vi "Find Object Items by Name.vi"(6 "Item Names":string[](array[string]), 7 "$Path or Item Name":string caption="Object $Path or Item Name", 8 "error in (no error)":errorcluster, 10 "Offset":i32, 11 "JSON":string) -> (0 "error out":errorcluster, 1 "<JSON>":string[](array[string]) caption="<JSON>Items", 2 "Offsets":i32[](array[numeric]))   [LabVIEW 2017, in "JSONtext.lvlib"]
doc: "Find multiple Items in a JSON Object, by item names. Output items (as JSON) are in the same order as the supplied item names. If an item is not present, then the output for that item will be an empty string."
uses:
  JSONtext.lvlib
  support/quote and escape json string 2.vi
  Offset/Find Item Locations by Path.vi
  Parsing/Parse Full Path or Item Name.vi
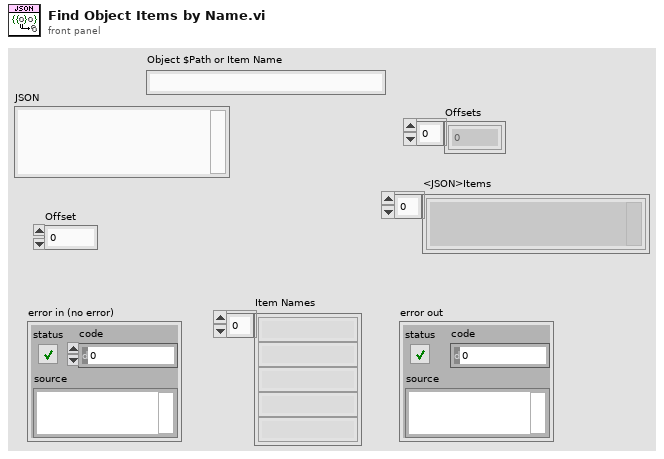
[diagram p1: front panel]
types:
  T1 = typedef "JSONtext.lvlib/Found Items.ctl" = cluster{"Item offset":i32, "Offset past Item":i32, "Name offset":i32, "Offset past Name":i32, "Found":bool, "Item Type":T2, "Item Index":i32}
  T2 = typedef "JSONtext.lvlib/Parsing State.ctl" = enum16{"Parser Error", "Object", "Array", "String", "Number/Other", "Leading Whitespace", "Object end", "Array end", "Value end"}
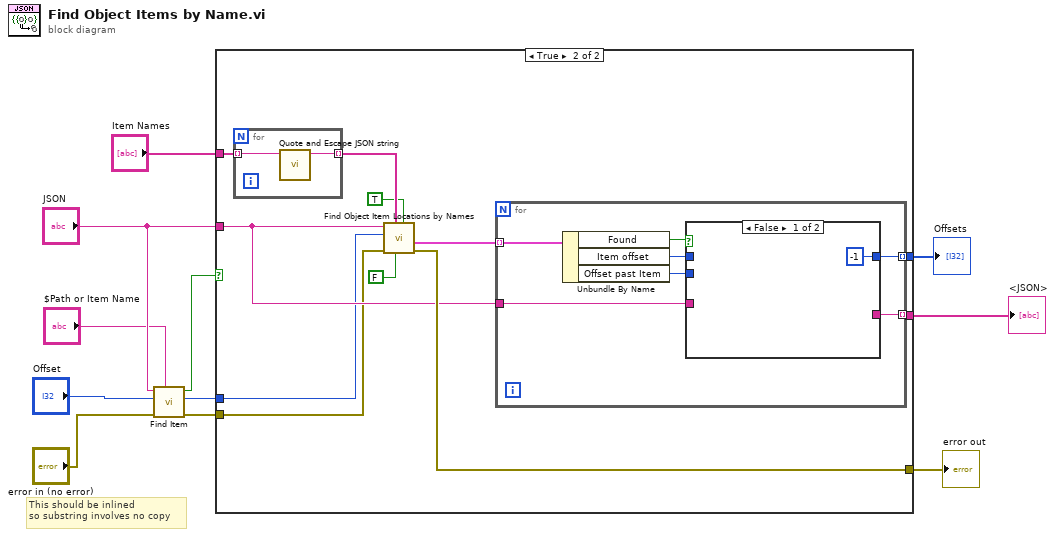
[diagram p0: block diagram]
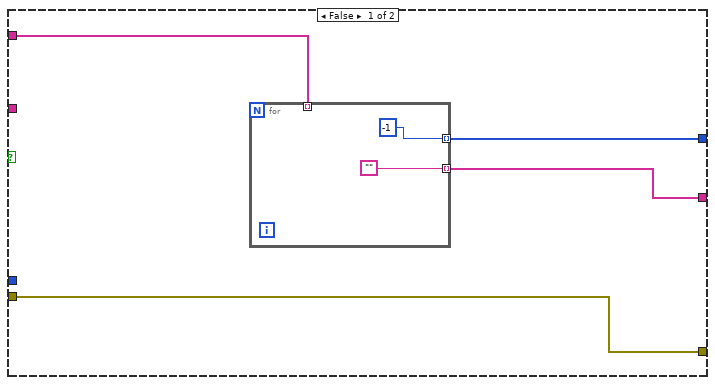
[diagram p2: hidden frame]
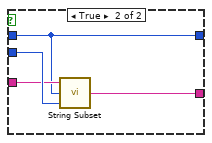
[diagram p3: hidden frame]
diagram:
  # "This should be inlined\nso substring involves no copy"
  n1 = call "Find Item.vi"("$Path or Item Name"="$Path or Item Name", "error in (no error)"="error in (no error)", "Offset"="Offset", "JSON"="JSON") -> ("error out"=w5:errorcluster, "Item offset"=w2:i32, "Found"=w4:bool)  [unwired: 4 in, 1 out]
  n2 = case shown="True" w4 {
    tunnel: [w15 w28] -> w11
    tunnel: [w13 w27] -> w10
    tunnel: "Item Names" -> [w14 w24]
    tunnel: "JSON" -> [_ w21]
    tunnel: w2 -> [_ w20]
    tunnel: w5 -> [w15 w19]
    tunnel: [w12 w18] -> w1
    frame False {
      n3 = for {
        tunnel: w14 -> [_] mode=indexing
        tunnel: [""] -> w13 mode=indexing
        tunnel: [-1] -> w12 mode=indexing
      }
    }
    frame True {
      n4 = for {
        tunnel: w24 -> [w30] mode=indexing
        tunnel: [w29] -> w23 mode=indexing
        n5 = call "Quote and Escape JSON string.vi"("Plain Text"=w30) -> ("<JSON>"=w29:string)  [unwired: 10 in]
      }
      n6 = call "Find Object Item Locations by Names.vi"("Insertion point if not found"=TRUE, "Only return first found"=FALSE, "Item Names <JSON>"=w23, "error in (no error)"=w19, "Object Offset"=w20, "JSON"=w21) -> ("error out"=w28:errorcluster, "Items"=w26:T1[])  [unwired: 4 in]
      n7 = for {
        tunnel: w21 -> [w37]
        tunnel: [w36] -> w27 mode=indexing
        tunnel: w26 -> [w33] mode=indexing
        tunnel: [w31] -> w18 mode=indexing
        n8 = Unbundle By Name(w33) -> ("Found"=w32:bool, "Item offset"=w35:i32, "Offset past Item"=w34:i32)
        n9 = case shown="False" w32 {
          tunnel: w37 -> [_ w40]
          tunnel: [_ w42] -> w36
          tunnel: w35 -> [_ w39]
          tunnel: w34 -> [_ w41]
          tunnel: [-1 ("Item offset") w39] -> w31
          frame False {
          }
          frame True {
            n10 = call "String Subset.vi"("Offset past End"=w41, "Start offset"=w39, "JSON"=w40) -> ("substring"=w42:string)  [unwired: 2 in]
          }
        }
      }
    }
  }
  "error out" <- w11
  "<JSON>" <- w10
  "Offsets" <- w1
